vi "Drive.vi"(8 "Drive R":dbl, 11 "Drive L":dbl) -> ()   [LabVIEW 2017]
uses:
  <vilib>/Rock Robotics/WPI/SafetyOutput/WPI_SafetyOutputConfigMenu.ctl
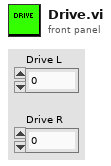
[diagram p1: front panel]
types:
  T1 = typedef "WPI_SafetyOutputConfigMenu.ctl" = enum16{"Enable", "Disable"}
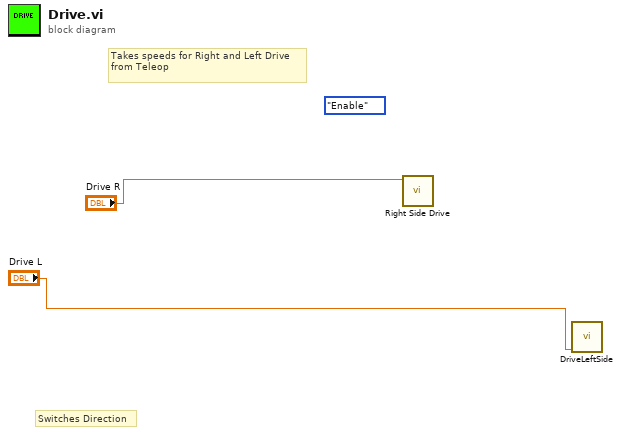
[diagram p0: block diagram]
diagram:
  (unwired) WPI_SafetyOutputConfigMenu."Enable" ("mode")
  # "Switches Direction"
  # "Takes speeds for Right and Left Drive\nfrom Teleop"
  n1 = call "Right Side Drive.vi"("Effort"="Drive R") -> ()  [unwired: 11 in]
  n2 = call "DriveLeftSide.vi"("Effort"="Drive L") -> ()  [unwired: 11 in]
